vi "DangerousToy.vi"() -> ()   [LabVIEW 2018]
uses:
  <vilib>/express/express analysis/Spectral/Block/exnSpectralBlock spectral measurements power poly.vi
  <vilib>/express/express analysis/Spectral/Block/exnSpectralBlock spectral measurements power DDT.vi
  <vilib>/express/express analysis/Spectral/XNode/ExpressSpectralMeasurementsBlockNode.xnode
  <vilib>/ptbypt/NI_PtbyPt.lvlib
panel:
  in  "stop":bool
  out "Waveform Graph":dynamicdata(graph)
  out "Signals":dynamicdata(graph)
  out "File Directory":path
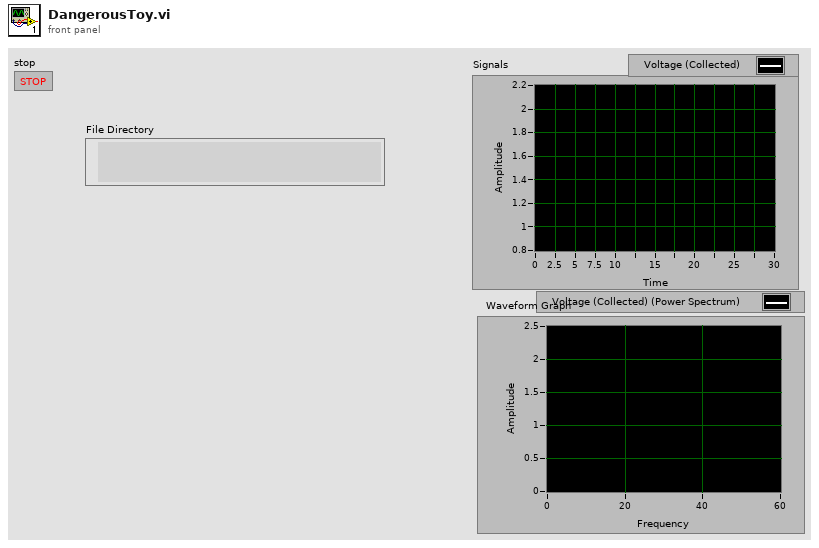
[diagram p1: front panel]
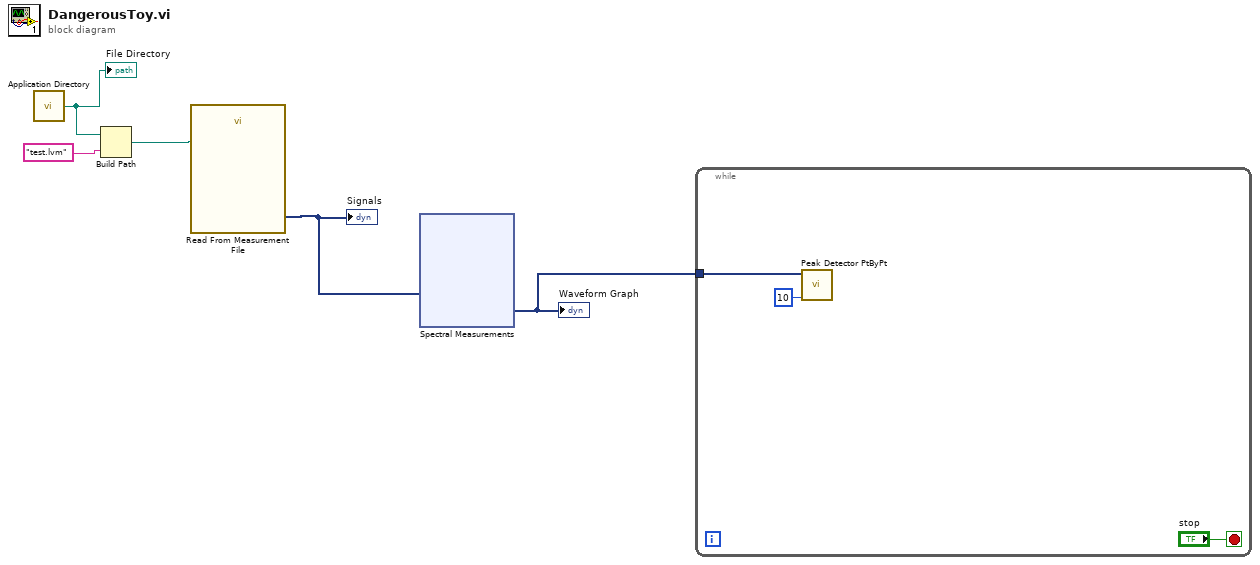
[diagram p0: block diagram]
diagram:
  n1 = call <vilib>:"Application Directory.vi"() -> ("Application Directory"=w5:path)
  "File Directory" <- w5
  n2 = Build Path(base path=w5, name or relative path="test.lvm") -> (appended path=w3:path)
  n3 = call "Read From Measurement File"("Filename"=w3) -> ("Signals"=w2:dynamicdata)  [unwired: 5 in, 5 out]
  "Signals" <- w2
  n4 = xnode "Spectral Measurements"("Signals"=w2) -> ("Power Spectrum"=w1:dynamicdata)  [unwired: 1 in, 1 out]
  "Waveform Graph" <- w1
  n5 = while {
    tunnel: w1 -> [w8]
    stop <- "stop" stop-if-true
    n6 = call <vilib>:"Peak Detector PtByPt.vi"("x"=w8, "width"=10) -> ()  [unwired: 3 in, 3 out]
  }
